vi "Close Bus Monitor.vi"(8 "error in (no error)":errorcluster, 11 "ListboxBusMonitor In":refnum<class "ListboxBusMonitor.lvclass">) -> (3 "ListboxBusMonitor Out":refnum<class "ListboxBusMonitor.lvclass">)   [LabVIEW 2020, in "MVA Framework.lvlib" / "ListboxBusMonitor.lvlib" / "ListboxBusMonitor.lvclass"]
doc: "关闭总线监视器"
uses:
  ListboxBusMonitor.lvclass
  <vilib>/ActorFramework/Message Enqueuer/Message Priority.ctl
  ListboxBusMonitor.lvclass/ListboxBusMonitor.ctl
  <vilib>/ActorFramework/Message Enqueuer/Message Enqueuer.lvclass/Message Enqueuer.ctl
  <vilib>/ActorFramework/Message Enqueuer/Enqueue.vi
  <vilib>/ActorFramework/Stop Msg/Stop Msg.lvclass
  C:/Program Files/National Instruments/LabVIEW 2020/vi.lib/ActorFramework/Message/Message.lvclass
  <vilib>/ActorFramework/Message Priority Queue/Priority Enqueue.vi
  modules/composed-af-messages/Source/PriorityStopMessage/PriorityStopMessage.lvclass
  <vilib>/ActorFramework/Message Enqueuer/Message Enqueuer.lvclass
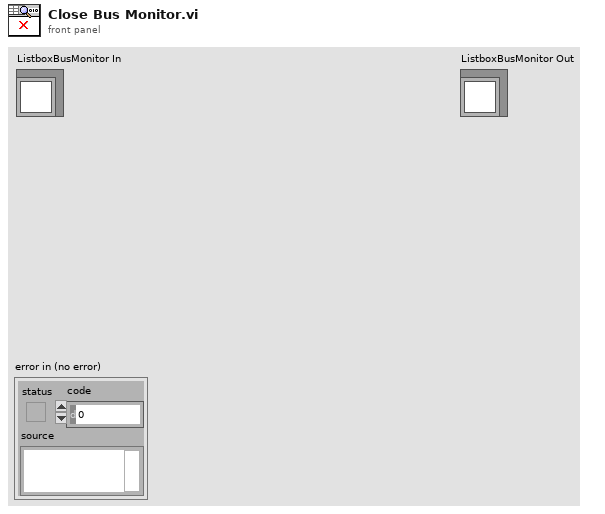
[diagram p1: front panel]
types:
  T1 = typedef "Actor Framework.lvlib/Message Enqueuer.lvclass/Message Priority.ctl" = enum16{"Low", "Normal", "High"}
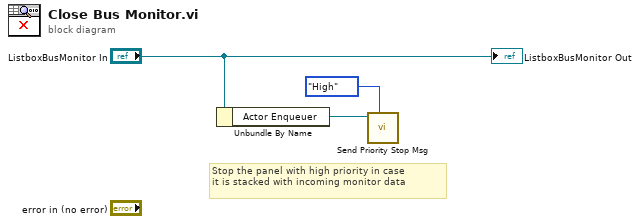
[diagram p0: block diagram]
diagram:
  # "Stop the panel with high priority in case\nit is stacked with incoming monitor data"
  n1 = Unbundle By Name("ListboxBusMonitor In") -> ("Actor Enqueuer"=w2:refnum<class "Message Enqueuer.lvclass">)
  n2 = call "Send Priority Stop Msg.vi"("Message Priority (Normal)"=Message_Priority."High", "Message Enqueuer"=w2) -> ()  [unwired: 9 in, 1 out]
  "ListboxBusMonitor Out" <- "ListboxBusMonitor In"
